vi "RS_generator_freq_powr.vi"(2 "Power (dBm)":dbl=-10.0 format="%#_13p", 3 "Frequnecy (Hz)":u64=100000) -> (0 "error out":errorcluster, 1 "resulting string":string)   [LabVIEW 2013]
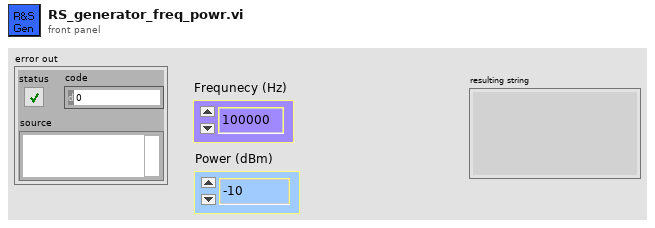
[diagram p1: front panel]
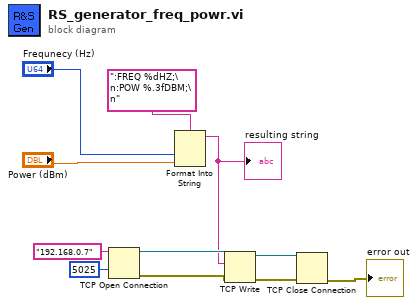
[diagram p0: block diagram]
diagram:
  n1 = TCP Open Connection(address="192.168.0.7", remote port or service name=u16 5025) -> (connection ID=w11:refnum<k5>, error out=w9:errorcluster)  [unwired: 3 in]
  n2 = Format Into String(format string=":FREQ %dHZ;\n:POW %.3fDBM;\n" ("string"), "Frequnecy (Hz)", "Power (dBm)") -> (resulting string=w4:string)  [unwired: 2 in, 1 out]
  "resulting string" <- w4
  n3 = TCP Write(connection ID=w11, data in=w4, error in (no error)=w9) -> (connection ID out=w10:refnum<k5>, error out=w8:errorcluster)  [unwired: 1 in, 1 out]
  n4 = TCP Close Connection(connection ID=w10, error in (no error)=w8) -> (error out=→"error out":errorcluster)  [unwired: 1 in, 1 out]
